vi "generateArray.vi"(10 "Cols":i32, 11 "Rows":i32) -> (3 "Array":dbl[][](array[numeric]))   [LabVIEW 2017]
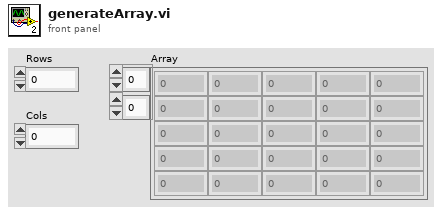
[diagram p1: front panel]
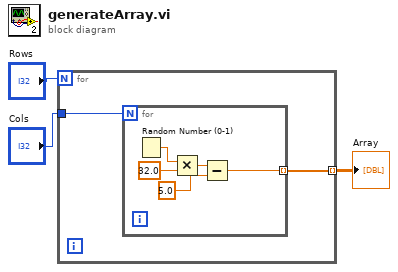
[diagram p0: block diagram]
diagram:
  n1 = for {
    N: "Rows" -> [_]
    tunnel: [w5] -> w2 mode=indexing
    tunnel: "Cols" -> [w4]
    n2 = for {
      N: w4 -> [_]
      tunnel: [w6] -> w5 mode=indexing
      n3 = Random Number (0-1)() -> (number: 0 to 1=w10:dbl)
      n4 = Multiply(x=w10, y=32.0) -> (x*y=w8:dbl)
      n5 = Subtract(x=w8, y=5.0) -> (x-y=w6:dbl)
    }
  }
  "Array" <- w2
